vi "Calculate Angle.vi"(8 "Pixel Divisor":dbl, 11 "Pixel In":dbl) -> (3 "Angle Out (Rad)":dbl)   [LabVIEW 2013]
panel:
  # "NOTE:  This will probably only be useful for Compute Distence.vi.\n\nHOWEVER, documentation is as follows.\n\nThis calculator may convert an X or Y coordinate from the camera\nto yaw or pitch from an imaginary line extending from the center of the camera,\nrespectively.\n\nCall with either X or Y coordinates; documentation assumes Y coordinates,\nmentally substitute with X as needed.\n\nPixel in:  Y coordinate of the pixel.\n\nPixel divisor:  Constant--do not set.  Calculate this with Calculate Resolution.vi.\n\nAngle Out (Rad):  Angle out in radians."
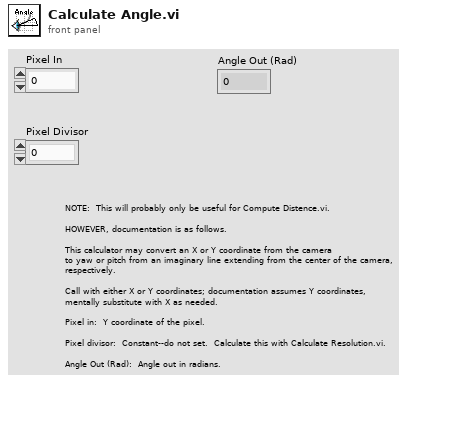
[diagram p1: front panel]
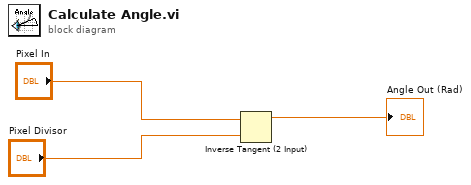
[diagram p0: block diagram]
diagram:
  n1 = Inverse Tangent (2 Input)(1:"Pixel Divisor", 2:"Pixel In") -> (0:→"Angle Out (Rad)":dbl)
